vi "GenerateWaveform.vi"(8 "error in (no error)":errorcluster, 11 "FunctionGenerator in":refnum<class "FunctionGenerator.lvclass">) -> (0 "error out":errorcluster, 3 "FunctionGenerator out":refnum<class "FunctionGenerator.lvclass">)   [LabVIEW 2020, in "FunctionGenerator.lvclass"]
uses:
  FunctionGenerator.lvclass
  C:/Code Projects/CircuitExplorer/AnalogDiscoveryFunction/AnalogDiscoveryFunction.lvclass
  AnalogDiscoveryFunction/AnalogDiscoveryFunction.lvclass/AnalogDiscoveryFunction.ctl
  AnalogDiscoveryFunction/GetInstrumentHandle.vi
  <vilib>/DigilentWF/DigilentWF.lvlib
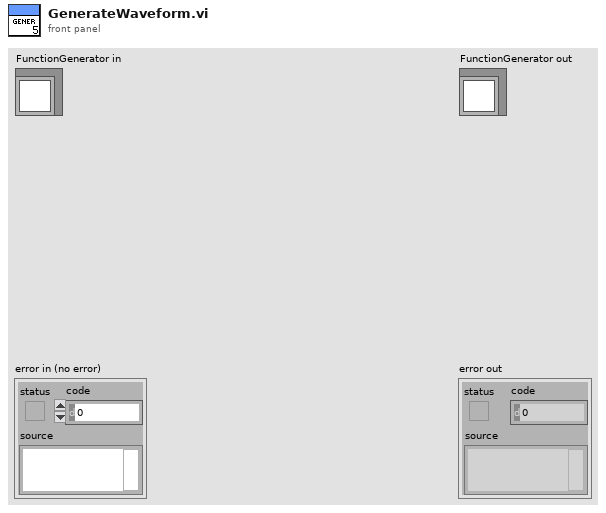
[diagram p1: front panel]
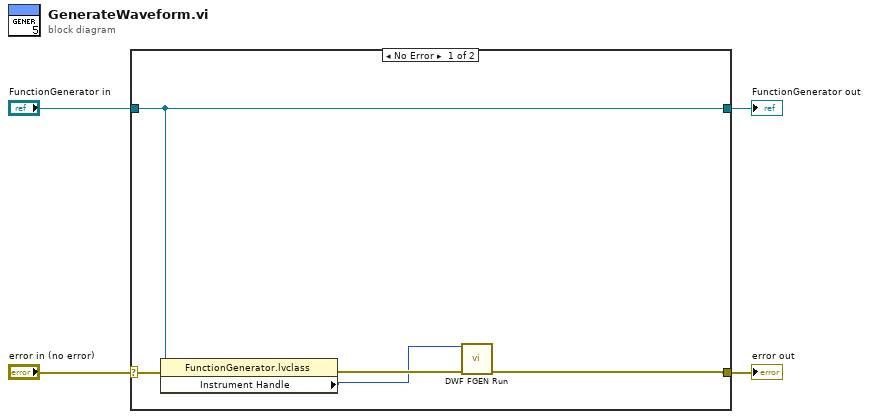
[diagram p0: block diagram]
diagram:
  n1 = case shown="No Error" "error in (no error)" {
    selector: "error in (no error)" -> [w9 w11]
    tunnel: [w6 w11] -> w3
    tunnel: [w8 w10] -> w1
    tunnel: "FunctionGenerator in" -> [w8 w10]
    frame No Error {
      n2 = property class="FunctionGenerator.lvclass"(reference=w8, error in=w9) -> (error out=w7:errorcluster, "Instrument Handle"=w5:u32)  [unwired: 1 out]
      n3 = call <vilib>:"DWF FGEN Run.vi"("Instrument Handle In"=w5, "Error In"=w7) -> ("Error Out"=w6:errorcluster)  [unwired: 12 in, 1 out]
    }
    frame Error {
    }
  }
  "error out" <- w3
  "FunctionGenerator out" <- w1
